vi "Publish X Axis.vi"(11 "X Axis":T1) -> ()   [LabVIEW 2016]
uses:
  <vilib>/Rock Robotics/Network Tables/NT Write Number.vi
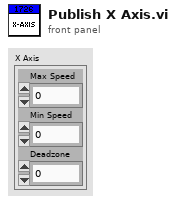
[diagram p1: front panel]
types:
  T1 = cluster{"Max Speed":dbl, "Min Speed":dbl, "Deadzone":dbl}
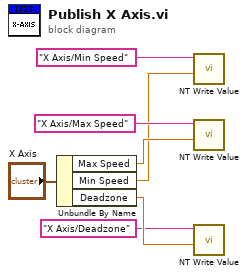
[diagram p0: block diagram]
diagram:
  n1 = Unbundle By Name("X Axis") -> ("Max Speed"=w7:dbl, "Min Speed"=w4:dbl, "Deadzone"=w5:dbl)
  n2 = call-poly <vilib>:"NT Write Value.vi"("Numeric"=w4, "Name"="X Axis/Min Speed") -> ()  [unwired: 9 in, 1 out]
  n3 = call-poly <vilib>:"NT Write Value.vi"("Numeric"=w7, "Name"="X Axis/Max Speed") -> ()  [unwired: 9 in, 1 out]
  n4 = call-poly <vilib>:"NT Write Value.vi"("Numeric"=w5, "Name"="X Axis/Deadzone") -> ()  [unwired: 9 in, 1 out]
